vi "KalmanFilterLatencyComp_Observer_New.vi"(8 "TimeStamp_Sec":dbl, 9 "LocalY":T2, 10 "U":T2, 11 "Observer":T1) -> (3 "OBSERVER_LIST_ITEM":T5)   [LabVIEW 2019, in "Trajectory_Library.lvlib"]
doc: "Creates the Observer List Item data cluster from individual input paramters.\n\nInputs:\n - observer -- The observer. (Uncented Kalman Filter) data cluster\n - u -- The input matrix at the timestamp.\n - localY -- The local output matrix at the timestamp\n - timestampSeconds -- The timesnap of the state.\n\nOutputs:\n - ObserverListItem -- Observer List Item data cluster (ready to push onto the list of stored items)"
uses:
  Trajectory_Library.lvlib
  TypeDef/OBSERVER_SNAP_LIST_ITEM.ctl
  TypeDef/OBSERVER_SNAPSHOT.ctl
  <vilib>/Analysis/Matrix/Datatypes/RealMatrix.ctl
  TypeDef/UNSCENTED_KALMAN_FILTER.ctl
  TypeDef/MERWE_SCALED_SIGMA_PTS.ctl
  TypeDef/CALLBACK_FUNC_TYPE.ctl
  <vilib>/Analysis/Matrix/NI_Matrix.lvlib
panel:
  # "State Estimate <Statess,1>"
  # "<States, States>"
  # "<States, ?>"
  # "<Statess,  States>"
  # "<Outputs, Outputs>"
  # "<?, 1>"
  # "<?, 1>"
  # "<Statess,1>"
  # "<States, States>"
  # "<Inputs, 1>"
  # "<Outputs,  1>"
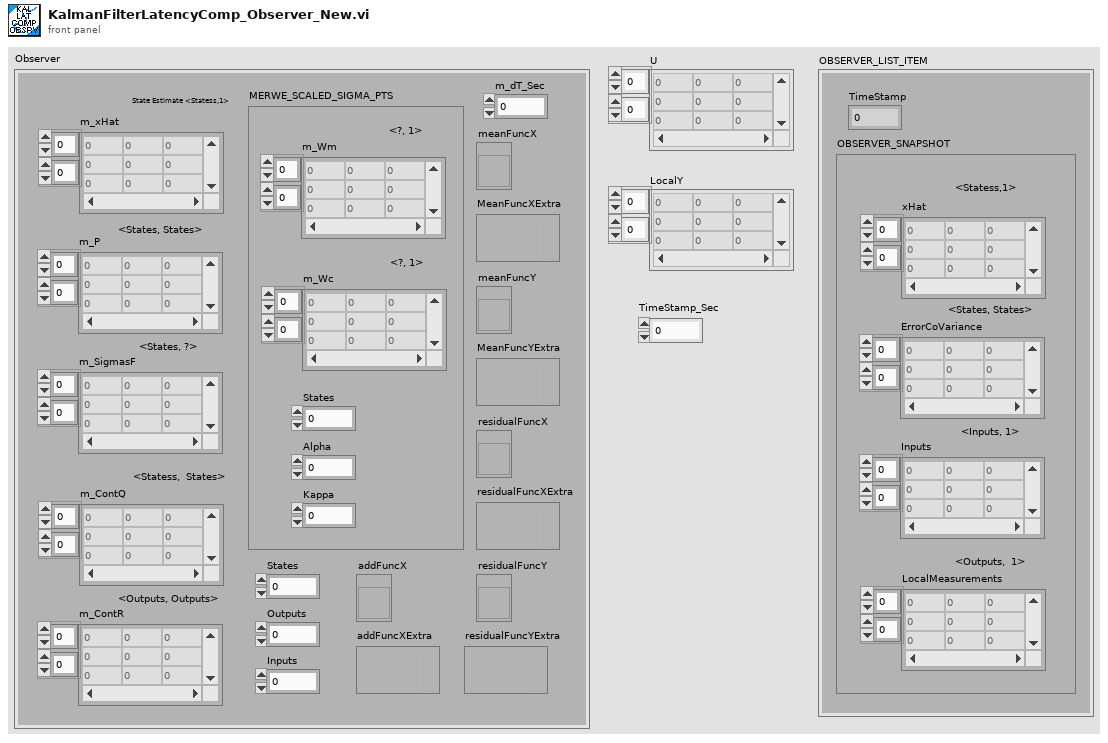
[diagram p1: front panel]
types:
  T1 = typedef "Trajectory_Library.lvlib/UNSCENTED_KALMAN_FILTER.ctl" = cluster{"m_P":T2, "m_xHat":T2, "States":i32, "Outputs":i32, "m_ContR":T2, "m_ContQ":T2, "m_SigmasF":T2, "m_dT_Sec":dbl, "MERWE_SCALED_SIGMA_PTS":T3, "meanFuncX":T4, "meanFuncY":T4, "residualFuncX":T4, "residualFuncY":T4, "addFuncX":T4, "addFuncXExtra":variant, "residualFuncYExtra":variant, "residualFuncXExtra":variant, "MeanFuncYExtra":variant, "MeanFuncXExtra":variant, "Inputs":i32}
  T2 = typedef "NI_Matrix.lvlib/RealMatrix.ctl" = dbl[][]
  T3 = typedef "Trajectory_Library.lvlib/MERWE_SCALED_SIGMA_PTS.ctl" = cluster{"m_Wm":T2, "States":i32, "Alpha":dbl, "m_Wc":T2, "Kappa":i32}
  T4 = typedef "Trajectory_Library.lvlib/CALLBACK_FUNC_TYPE.ctl" = refnum<vi>
  T5 = typedef "Trajectory_Library.lvlib/OBSERVER_SNAP_LIST_ITEM.ctl" = cluster{"TimeStamp":dbl, "OBSERVER_SNAPSHOT":T6}
  T6 = typedef "Trajectory_Library.lvlib/OBSERVER_SNAPSHOT.ctl" = cluster{"ErrorCoVariance":T2, "xHat":T2, "LocalMeasurements":T2, "Inputs":T2}
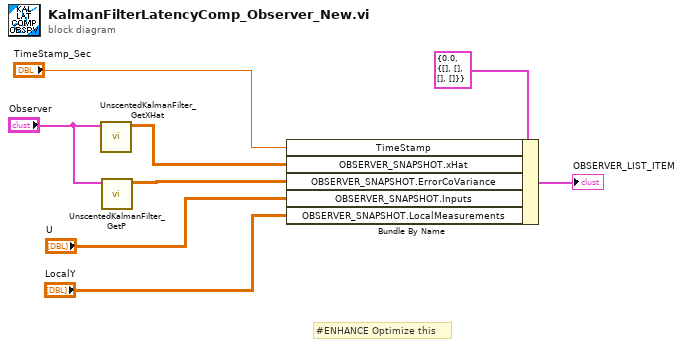
[diagram p0: block diagram]
diagram:
  # "#ENHANCE Optimize this"
  n1 = call "UnscentedKalmanFilter_GetXHat.vi"("in UnscentedKalmanFiilter"="Observer") -> ("xHat"=w3:T2)  [unwired: 10 in]
  n2 = call "UnscentedKalmanFilter_GetP.vi"("in UnscentedKalmanFiilter"="Observer") -> ("P"=w2:T2)  [unwired: 10 in]
  n3 = Bundle By Name(cluster=T5 {"TimeStamp"=0.0, "OBSERVER_SNAPSHOT"={"ErrorCoVariance"=[], "xHat"=[], "LocalMeasurements"=[], "Inputs"=[]}} ("OBSERVER_LIST_ITEM"), "TimeStamp"="TimeStamp_Sec", "OBSERVER_SNAPSHOT.xHat"=w3, "OBSERVER_SNAPSHOT.ErrorCoVariance"=w2, "OBSERVER_SNAPSHOT.Inputs"="U", "OBSERVER_SNAPSHOT.LocalMeasurements"="LocalY") -> (→"OBSERVER_LIST_ITEM":T5)
